vi "INIHandle.vi"(2 "Mode":enum16{"INIT", "OWC", "ORC"}(ring), 5 "VI Refnum":refnum<vi>, 11 "error in (no error)":errorcluster) -> (15 "error out":errorcluster)   [LabVIEW 2011]
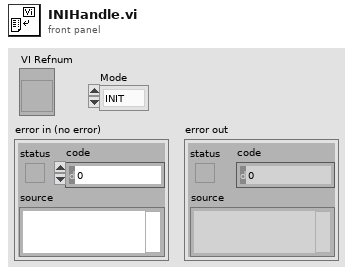
[diagram p1: front panel]
types:
  T1 = enum16{"Refnum", "Open", "Read", "Write", "Close"}
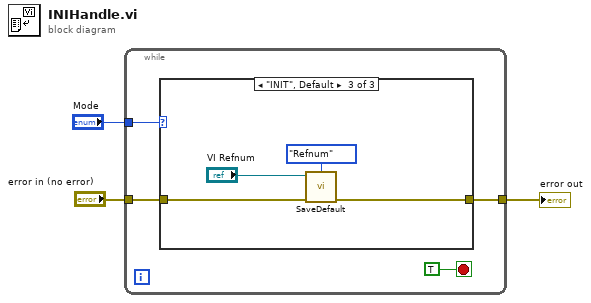
[diagram p0: block diagram]
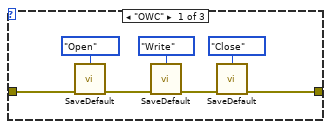
[diagram p2: hidden frame]
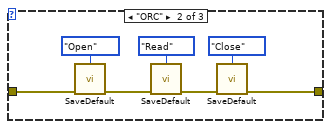
[diagram p3: hidden frame]
diagram:
  n1 = while {
    tunnel: "Mode" -> [w6]
    tunnel: "error in (no error)" -> [w5]
    tunnel: [w4] -> w1
    stop <- TRUE stop-if-true
    n2 = case shown="\"INIT\", Default" w6 {
      tunnel: w5 -> [w11 w18 w24]
      tunnel: [w8 w15 w23] -> w4
      frame "OWC" {
        n3 = call "SaveDefault.vi"("Mode"=T1."Open", "error in (no error)"=w11) -> ("error out"=w10:errorcluster)  [unwired: 13 in]
        n4 = call "SaveDefault.vi"("Mode"=T1."Write", "error in (no error)"=w10) -> ("error out"=w9:errorcluster)  [unwired: 13 in]
        n5 = call "SaveDefault.vi"("Mode"=T1."Close", "error in (no error)"=w9) -> ("error out"=w8:errorcluster)  [unwired: 13 in]
      }
      frame "ORC" {
        n6 = call "SaveDefault.vi"("Mode"=T1."Open", "error in (no error)"=w18) -> ("error out"=w17:errorcluster)  [unwired: 13 in]
        n7 = call "SaveDefault.vi"("Mode"=T1."Read", "error in (no error)"=w17) -> ("error out"=w16:errorcluster)  [unwired: 13 in]
        n8 = call "SaveDefault.vi"("Mode"=T1."Close", "error in (no error)"=w16) -> ("error out"=w15:errorcluster)  [unwired: 13 in]
      }
      frame "INIT", Default {
        n9 = call "SaveDefault.vi"("VI Refnum"="VI Refnum", "Mode"=T1."Refnum", "error in (no error)"=w24) -> ("error out"=w23:errorcluster)  [unwired: 12 in]
      }
    }
  }
  "error out" <- w1
